vi "pb_write_three.vi"(1 "error in (no error)":errorcluster, 2 "8-bit data":u32, 3 "8-bit address offset":u32) -> (0 "error out":errorcluster)   [LabVIEW 2013, in "PulseBlaster.lvlib"]
uses:
  PulseBlaster.lvlib
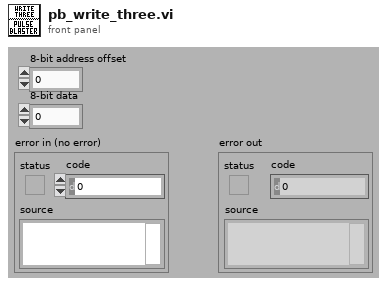
[diagram p1: front panel]
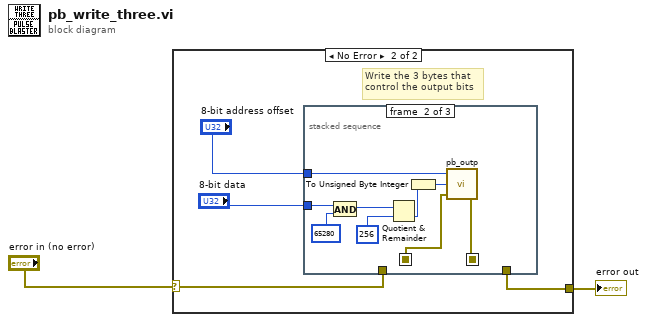
[diagram p0: block diagram]
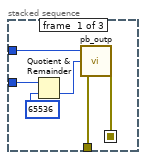
[diagram p3: hidden frame]
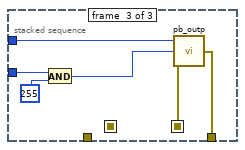
[diagram p4: hidden frame]
diagram:
  n1 = case shown="No Error" "error in (no error)" {
    selector: "error in (no error)" -> [w3 w5]
    tunnel: [w3 w4] -> w1
    frame Error {
    }
    frame No Error {
      # "Write the 3 bytes that \ncontrol the output bits"
      n2 = stacked-sequence {
        seq-local: [w8 _ _] -> [_ w15 _]
        seq-local: [_ w14 _] -> [_ _ w24]
        tunnel: "8-bit data" -> [w12 w20 w27]
        tunnel: "8-bit address offset" -> [w10 w17 w26]
        tunnel: w5 -> [w9 _ _]
        tunnel: [_ _ w23] -> w4
        frame #0 {
          n3 = Quotient & Remainder(x=w12, y=u32 65536) -> (floor(x/y)=w11:u32)  [unwired: 1 out]
          n4 = call "pb_outp.vi"("error in (no error)"=w9, "8-bit data"=w11, "8-bit address offset"=w10) -> ("error out"=w8:errorcluster)
        }
        frame #1 {
          n5 = And(x=w20, y=u32 65280) -> (x .and. y?=w19:u32)
          n6 = Quotient & Remainder(x=w19, y=u32 256) -> (floor(x/y)=w18:u32)  [unwired: 1 out]
          n7 = To Unsigned Byte Integer(number=w18) -> (unsigned 8bit integer=w16:u8)
          n8 = call "pb_outp.vi"("error in (no error)"=w15, "8-bit data"=w16, "8-bit address offset"=w17) -> ("error out"=w14:errorcluster)
        }
        frame #2 {
          n9 = And(x=w27, y=u32 255) -> (x .and. y?=w25:u32)
          n10 = call "pb_outp.vi"("error in (no error)"=w24, "8-bit data"=w25, "8-bit address offset"=w26) -> ("error out"=w23:errorcluster)
        }
      }
    }
  }
  "error out" <- w1
